vi "Program Start.vi"() -> (0 "error out":errorcluster, 2 "Class Objects":T1, 3 "user events":refnum<queue>, 4 "user interface":refnum<queue>, 5 "Event Registration Refnum out":refnum<event-registration>, 7 "user event":refnum<user-event>)   [LabVIEW 2011]
uses:
  Controls/User Interface Control.ctl
  Controls/User Interface Action.ctl
  Controls/Class Objects.ctl
  Modules/File/Configuration/Configuration.lvclass
  Modules/Hardware/Power Supply/Power Supply.lvclass
  Modules/Hardware/Mass Flow Controller/Mass Flow Controller.lvclass
  Modules/Hardware/Detector/Detector.lvclass
  Modules/File/TDMS/TDMS.lvclass
  Controls/User Event Control.ctl
  Controls/User Event Action.ctl
  Functional Globals/User Interface Global Action.ctl
  Error Handling/Error Module Action.ctl
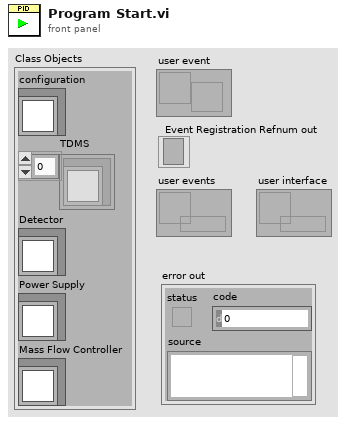
[diagram p1: front panel]
types:
  T1 = typedef "Class Objects.ctl" = cluster{"configuration":refnum<class "Configuration.lvclass">, "TDMS":refnum<class "TDMS.lvclass">[], "Power Supply":refnum<class "Power Supply.lvclass">, "Mass Flow Controller":refnum<class "Mass Flow Controller.lvclass">, "Detector":refnum<class "Detector.lvclass">}
  T2 = typedef "Error Module Action.ctl" = enum16{"Initialize", "Handle Errors", "Report Errors"}
  T3 = typedef "User Interface Global Action.ctl" = enum16{"Initialize", "Update UI", "Stop"}
  T4 = typedef "User Interface Control.ctl" = cluster{"action":T5, "data1":variant, "data2":variant}
  T5 = typedef "User Interface Action.ctl" = enum16{"Initialize", "Visibility Front Panel Controls", "Stop"}
  T6 = typedef "User Event Control.ctl" = cluster{"action":T7, "data":variant}
  T7 = typedef "User Event Action.ctl" = enum16{"Initialize", "Device Connections", "Device Settings", "Shutdown"}
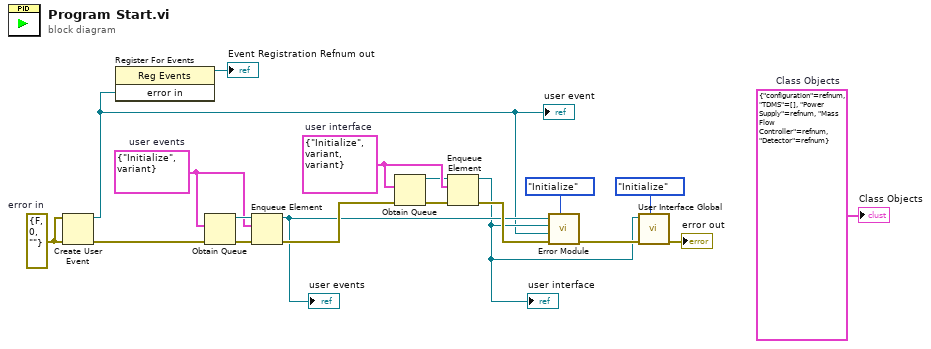
[diagram p0: block diagram]
diagram:
  w18 = T1 {"configuration"=refnum, "TDMS"=[], "Power Supply"=refnum, "Mass Flow Controller"=refnum, "Detector"=refnum}  # Class Objects
  w17 = T4 {"action"=enum."Initialize", "data1"=variant, "data2"=variant}  # user interface
  w12 = T6 {"action"=enum."Initialize", "data"=variant}  # user events
  w19 = errorcluster {"status"=FALSE, "code"=0, "source"=""}  # error in
  n1 = Create User Event(user event datatype=w19, error in=w19) -> (user event=w1:refnum<user-event>, error out=w16:errorcluster)
  "user event" <- w1
  n2 = register-events(w1) -> (reference out=→"Event Registration Refnum out":refnum<event-registration>)  [unwired: 2 in, 1 out]
  n3 = Obtain Queue(element data type=w12, error in (no error)=w16) -> (queue out=w13:refnum<queue>, error out=w11:errorcluster)  [unwired: 3 in, 1 out]
  n4 = Enqueue Element(queue=w13, element=w12, error in (no error)=w11) -> (queue out=w4:refnum<queue>, error out=w6:errorcluster)  [unwired: 1 in, 1 out]
  "user events" <- w4
  n5 = Obtain Queue(element data type=w17, error in (no error)=w6) -> (queue out=w15:refnum<queue>, error out=w14:errorcluster)  [unwired: 3 in, 1 out]
  n6 = Enqueue Element(queue=w15, element=w17, error in (no error)=w14) -> (queue out=w3:refnum<queue>, error out=w5:errorcluster)  [unwired: 1 in, 1 out]
  "user interface" <- w3
  n7 = call "Error Module.vi"("Command (Handle Errors"=Error_Module_Action."Initialize", "error in"=w5, "dynamic event queue reference"=w1, "User Interface Queue Reference"=w3, "User Event Queue Refence"=w4) -> ("error out"=w7:errorcluster)  [unwired: 5 in, 1 out]
  n8 = call "User Interface Global.vi"("command"=User_Interface_Global_Action."Initialize" ("Command (Update UI)"), "error in"=w7, "user interface"=w3) -> ("error out"=→"error out":errorcluster)  [unwired: 8 in]
  "Class Objects" <- w18
